vi "set_map.vi"(3 "error in":errorcluster, 4 "Map":string="Almono", 5 "Simulator Configuration in":string) -> (0 "error out":errorcluster, 2 "Simulator Configuration out":string)   [LabVIEW 2019, in "Lib_Simx.lvlib"]
doc: "Replaces the map name on the *Simulator configuration* with the specified map on the *Map* input"
uses:
  Lib_Simx.lvlib
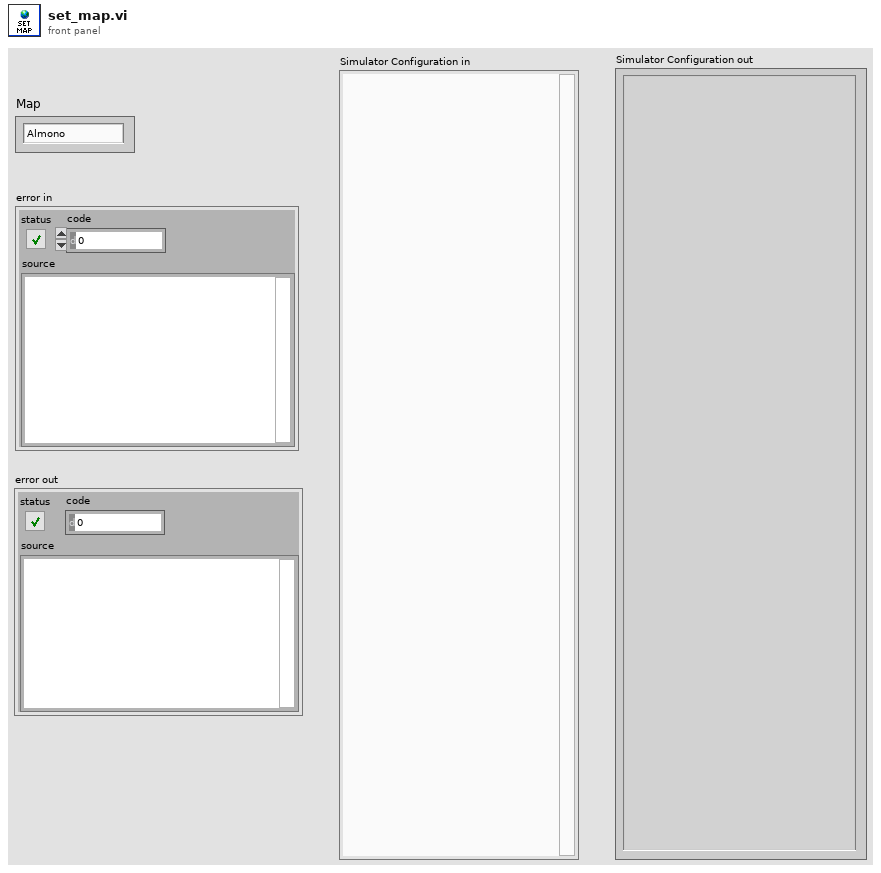
[diagram p1: front panel]
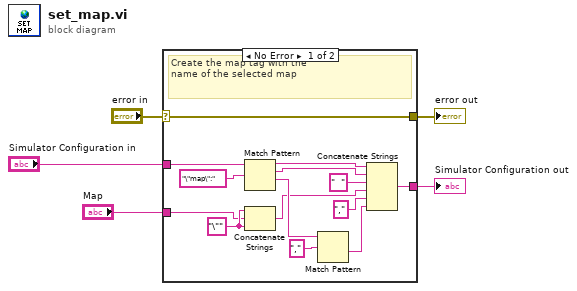
[diagram p0: block diagram]
diagram:
  n1 = case shown="No Error" "error in" {
    selector: "error in" -> [w7 w21]
    tunnel: [w7 w21] -> w4
    tunnel: "Simulator Configuration in" -> [w13 w20]
    tunnel: [w12 w20] -> w2
    tunnel: "Map" -> [w6 _]
    frame No Error {
      w9 = "\"" ("string")
      # "Create the map tag with the\nname of the selected map"
      n2 = Match Pattern(string=w13, regular expression="\"map\":" ("search string")) -> (before substring=w16:string, match substring=w15:string, after substring=w18:string)  [unwired: 1 in, 1 out]
      n3 = Concatenate Strings(w9, w6, w9) -> (w8:string)
      n4 = Match Pattern(string=w18, regular expression=",") -> (after substring=w11:string)  [unwired: 1 in, 3 out]
      n5 = Concatenate Strings(w16, w15, "  " ("string"), w8, "," ("string"), w11) -> (w12:string)
    }
    frame Error {
    }
  }
  "error out" <- w4
  "Simulator Configuration out" <- w2
